vi "create Server.vi"(11 "pServerId":i32) -> (3 "function return":i32)   [LabVIEW 2012, in "cvlib.lvlib"]
doc: "extern \"C\" __declspec(dllexport) long __cdecl createServer( long pServerId);"
uses:
  cvlib.lvlib
  build/labview/lvcvlib/cvlib.dll
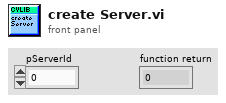
[diagram p1: front panel]
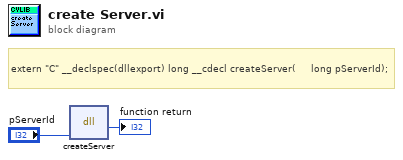
[diagram p0: block diagram]
diagram:
  # "extern \"C\" __declspec(dllexport) long __cdecl createServer(\t\t\t\t\tlong pServerId);"
  n1 = dll-call lib="C:/Users/myerslab/workspace2/Libraries/ClearVolume/build/labview/lvcvlib/cvlib.*" fn="createServer"("pServerId"="pServerId") -> (→"function return":i32)  [unwired: 4 in, 2 out]
